vi "组件表-累积功能管理表.vi"(8 "引用-累积功能管理列表":refnum<vi>, 9 "error in (no error)":errorcluster, 11 "DB 引用":T1) -> (0 "error out":errorcluster, 3 "数据库连接引用 o":T1, 4 "引用-累积功能管理表 o":refnum<vi>)   [LabVIEW 2017]
uses:
  <vilib>/addons/database/Connection.llb/Conn ObjectReference.ctl
  <vilib>/addons/database/NI_Database_API.lvlib
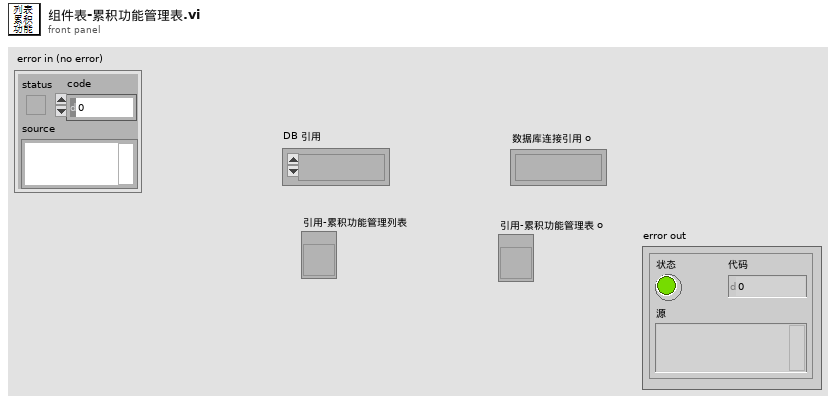
[diagram p1: front panel]
types:
  T1 = typedef "NI_Database_API.lvlib/Conn ObjectReference.ctl" = refnum<k1>
  T2 = cluster{"设备名称":string, "启用累积？":bool, "起始时间":timestamp, "累积剂量":dbl, "累积报警阈值":dbl}[]
  T3 = cluster{"设备名称":string, "启用累积？":bool, "起始时间":timestamp, "累积剂量":dbl, "累积报警阈值":dbl}
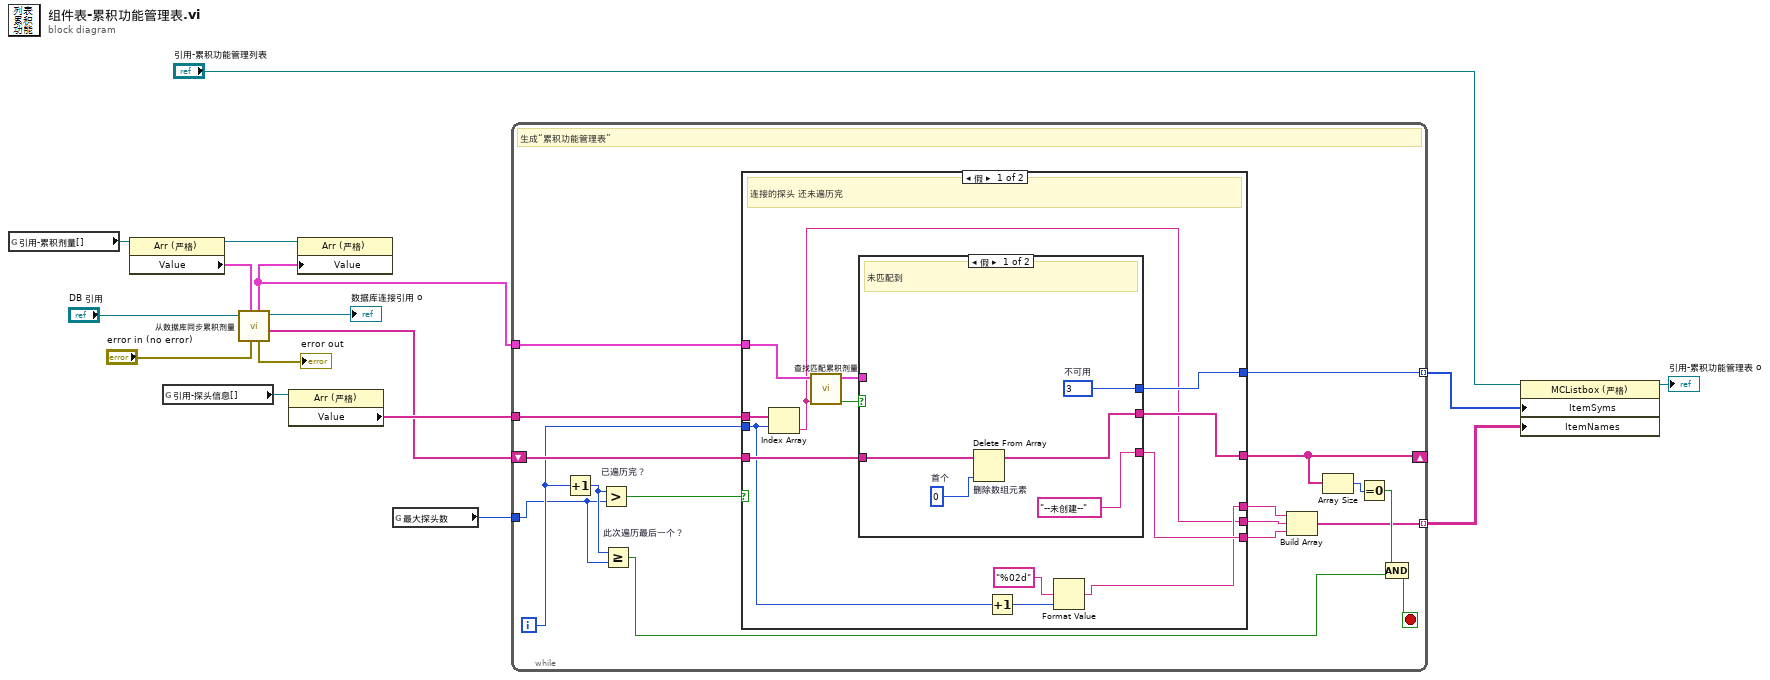
[diagram p0: block diagram]
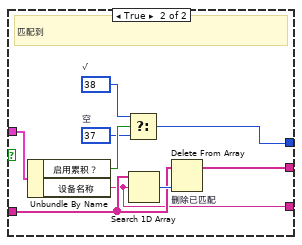
[diagram p2: hidden frame]
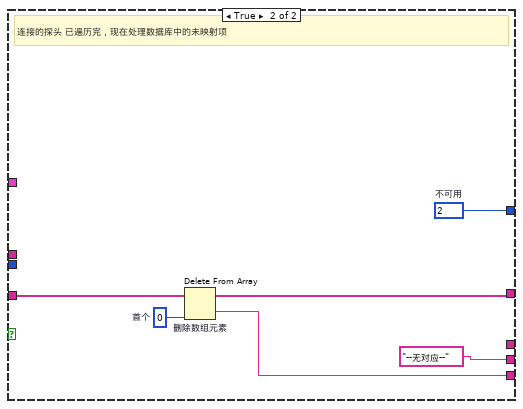
[diagram p3: hidden frame]
diagram:
  n1 = global read "全局变量-35点监测.vi" "引用-累积剂量[]"() -> (w9:refnum<vi>)
  n2 = property class="Arr (严格)"(reference=w9) -> (reference out=w8:refnum<vi>, "Value"=w4:T2)  [unwired: 1 in, 1 out]
  n3 = global read "全局变量-35点监测.vi" "引用-探头信息[]"() -> (w13:refnum<vi>)
  n4 = call "从数据库同步累积剂量.vi"("error in (no error)"="error in (no error)", "累积剂量 i"=w4, "数据库连接引用 i"="DB 引用") -> ("表名"=w7:string[], "数据库连接引用 o"=→"数据库连接引用 o":T1, "error out"=→"error out":errorcluster, "累积剂量 o"=w1:T2)  [unwired: 5 in]
  n5 = property class="Arr (严格)"(reference=w13) -> ("Value"=w14:string[])  [unwired: 1 in, 2 out]
  n6 = property class="Arr (严格)"(reference=w8, "Value"=w1) -> ()  [unwired: 1 in, 2 out]
  n7 = global read "全局变量-35点监测.vi" "最大探头数"() -> (w10:i32)
  n8 = while {
    tunnel: w1 -> [w29]
    tunnel: [w33] -> w15 mode=indexing
    shift-right: [w28] -> _
    shift-left: w7 -> [w32]
    tunnel: w10 -> [w18]
    tunnel: w14 -> [w31]
    tunnel: [w22] -> w16 mode=indexing
    i -> [w30]
    stop <- w21 stop-if-true
    # "生成“累积功能管理表”"
    n9 = Increment(x=w30) -> (x+1=w19:i32)
    n10 = Greater? "已遍历完？"(x=w19, y=w18) -> (0:w20:bool)
    n11 = Greater Or Equal? "此次遍历最后一个？"(x=w19, y=w18) -> (x >= y?=w17:bool)
    n12 = case shown="假" w20 {
      tunnel: [w46 w66] -> w33
      tunnel: [w34 "--无对应--" ("SQL query")] -> w24
      tunnel: w32 -> [w45 w64]
      tunnel: [w44 w63] -> w28
      tunnel: w31 -> [w43 _]
      tunnel: w30 -> [w39 _]
      tunnel: w29 -> [w42 _]
      tunnel: [w35 _] -> w25
      tunnel: [w38 w61] -> w23
      frame False {
        # "连接的探头 还未遍历完"
        n13 = Index Array(array=w43, index=w39) -> (element=w34:string)
        n14 = call "查找匹配累积剂量.vi"("探头名称"=w34, "累积剂量"=w42) -> ("匹配？"=w41:bool, "匹配的累积剂量"=w40:T3)  [unwired: 7 in, 1 out]
        n15 = case shown="假" w41 {
          tunnel: [w51 w57] -> w46
          tunnel: w45 -> [w50 w55]
          tunnel: [w49 w54] -> w44
          tunnel: w40 -> [_ w53]
          tunnel: ["--未创建--" ("设备名称") w52] -> w38
          frame False {
            w48 = 0  # 首个
            w51 = 3  # 不可用
            # "未匹配到"
            n16 = Delete From Array "删除数组元素"(array=w50, index=w48) -> (array with subset deleted=w49:string[])  [unwired: 1 in, 1 out]
          }
          frame True {
            w59 = 37  # 空
            w58 = 38  # √
            # "匹配到"
            n17 = Unbundle By Name(w53) -> ("启用累积？"=w60:bool, "设备名称"=w52:string)
            n18 = Select(t=w58, s=w60, f=w59) -> (s? t:f=w57:i32)
            n19 = Search 1D Array(1D array=w55, element=w52) -> (index of element=w56:i32)  [unwired: 1 in]
            n20 = Delete From Array "删除已匹配"(array=w55, index=w56) -> (array with subset deleted=w54:string[])  [unwired: 1 in, 1 out]
          }
        }
        n21 = Increment(x=w39) -> (x+1=w37:i32)
        n22 = Format Value(format string="%02d" ("格式字符串"), value (0)=w37) -> (output string=w35:string)  [unwired: 1 in]
      }
      frame True {
        w65 = 0  # 首个
        w66 = 2  # 不可用
        # "连接的探头 已遍历完，现在处理数据库中的未映射项"
        n23 = Delete From Array "删除数组元素"(array=w64, index=w65) -> (deleted portion=w61:string, array with subset deleted=w63:string[])  [unwired: 1 in]
      }
    }
    n24 = Build Array(w25, w24, w23) -> (w22:string[])
    n25 = Array Size(array=w28) -> (size(s)=w27:i32)
    n26 = Equal To 0?(x=w27) -> (x = 0?=w26:bool)
    n27 = Compound Arithmetic op=AND(w26, w17) -> (w21:bool)
  }
  n28 = property on="属性节点" class="MCListbox (严格)"(reference="引用-累积功能管理列表", "ItemSyms"=w15, "ItemNames"=w16) -> (reference out=→"引用-累积功能管理表 o":refnum<vi>)  [unwired: 1 in, 1 out]
